vi "Data Graph.vi"() -> ()   [LabVIEW 2013]
panel:
  out "XY Graph":cluster{"X":dbl, "Y":dbl}[](graph)
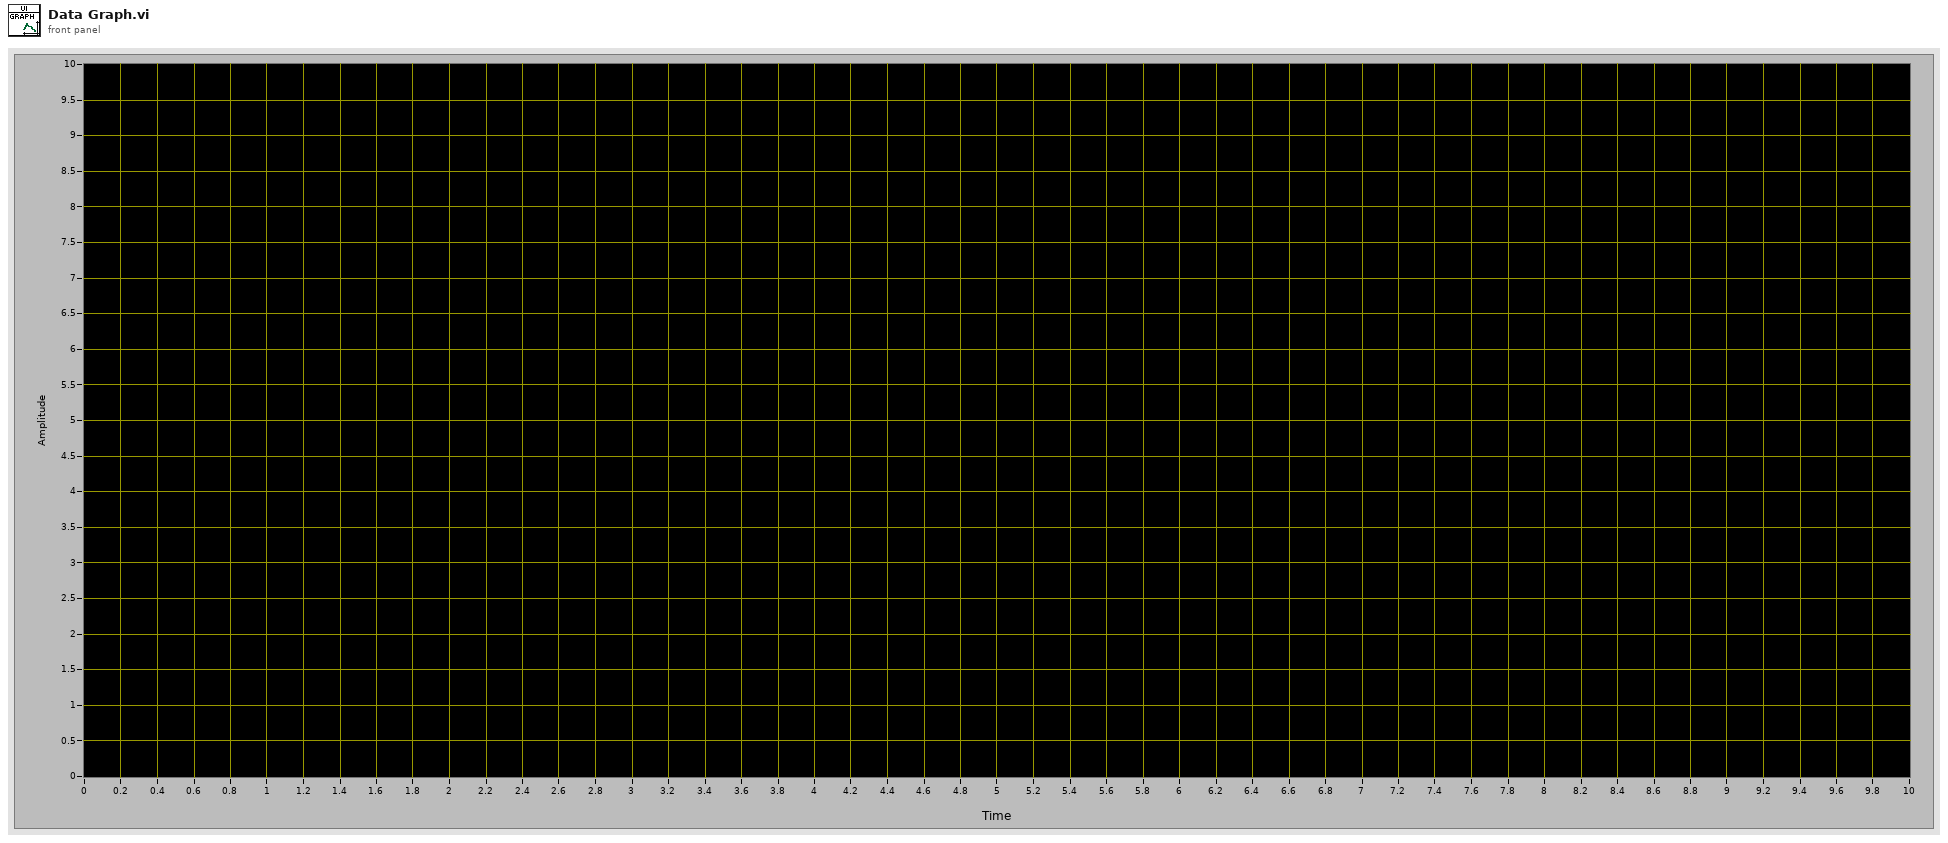
[diagram p1: front panel]
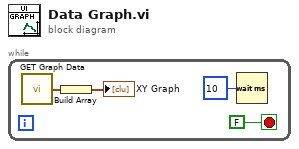
[diagram p0: block diagram]
diagram:
  n1 = while {
    stop <- FALSE stop-if-true
    n2 = call "GET Graph Data.vi"() -> ("Graph Data"=w4:cluster{"X":dbl, "Y":dbl})
    n3 = Build Array(w4) -> (→"XY Graph":cluster{"X":dbl, "Y":dbl}[])
    n4 = Wait (ms)(milliseconds to wait=u32 10) -> ()  [unwired: 1 out]
  }
